vi "Context to State.vi"(8 "error in":errorcluster, 10 "Context in":refnum<class "State Pattern.lvclass">) -> (0 "error out":errorcluster, 3 "State out":refnum<class "State Pattern.lvclass">, 5 "Context out (for Preserve Run-Time Class)":refnum<class "State Pattern.lvclass">)   [LabVIEW 2021, in "State Pattern.lvclass"]
uses:
  State Pattern.lvclass
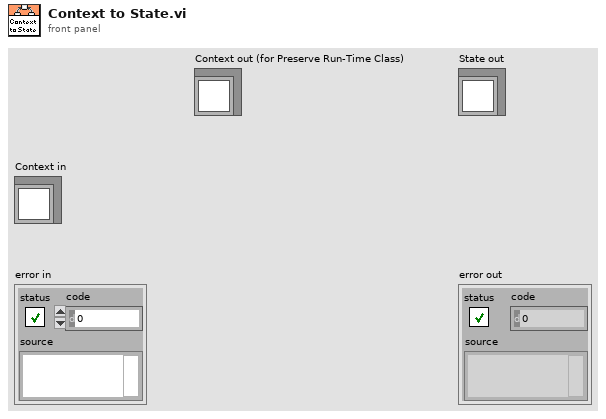
[diagram p1: front panel]
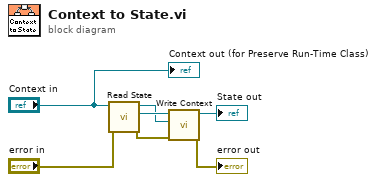
[diagram p0: block diagram]
diagram:
  n1 = call-dynamic "Read State.vi"("error in"="error in", "Context in"="Context in") -> ("error out"=w3:errorcluster, "State"=w5:refnum<class "State Pattern.lvclass">, "Context out"=w4:refnum<class "State Pattern.lvclass">)  [unwired: 7 in]
  n2 = call-dynamic "Write Context.vi"("error in"=w3, "Context"=w4, "State in"=w5) -> ("error out"=→"error out":errorcluster, "State out"=→"State out":refnum<class "State Pattern.lvclass">)  [unwired: 7 in]
  "Context out (for Preserve Run-Time Class)" <- "Context in"
